vi "Matrix - Complex.vi"(5 "use temporary file?":bool, 7 "data type of variable":cdb[][](array[numeric]), 8 "error in":errorcluster, 10 "variable name":string, 11 "pipe in":T1) -> (0 "error out":errorcluster, 2 "value":cdb[][](array[numeric]) format="%.2f", 3 "pipe out":T1)   [LabVIEW 2013, in "GOLPI library.lvlib"]
uses:
  GOLPI library.lvlib
  LV Process.lvlibp/Pipe Handle.ctl
  Custom Error Codes Enum Type Def.vi
  LV Process.lvlibp
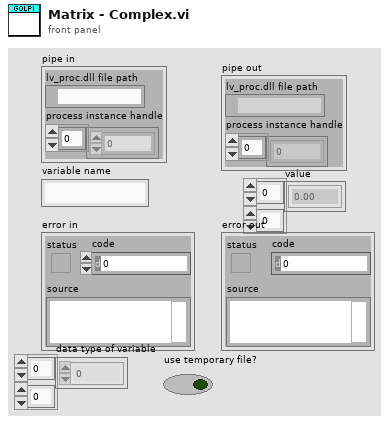
[diagram p1: front panel]
types:
  T1 = typedef "LV Process.lvlibp/Pipe Handle.ctl" = cluster{"lv_proc.dll file path":path, "process instance handle":u32[]}
  T2 = typedef "GOLPI library.lvlib/Custom Error Codes Enum Type Def.vi" = enum16{"no error", "00 working directory PAR1 missing", "01 octave binary PAR1 missing", "02 octave report error PAR1", "03 empty output last cmd PAR1", "04 missing temporary file PAR1", "10 var PAR1 not string", "11 var PAR1 not num, scal, ~compl", "12 var PAR1 not num, scal, compl", "13 var PAR1 not num, vect, ~compl", "14 var PAR1 not num, vect, compl", "15 var PAR1 not num, mat, ~compl", "16 var PAR1 not num, mat, ~compl", "99 not finished"}
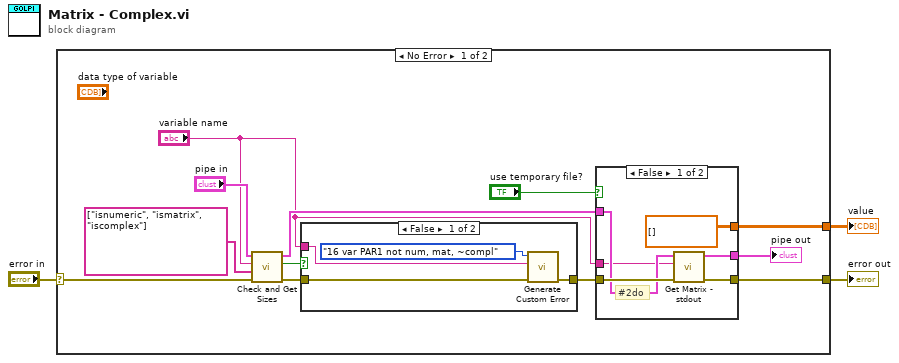
[diagram p0: block diagram]
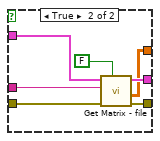
[diagram p2: hidden frame]
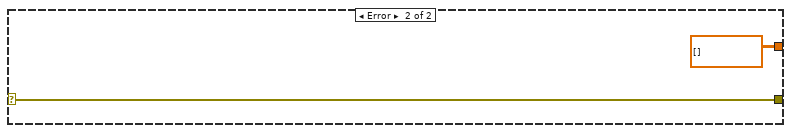
[diagram p4: hidden frame]
diagram:
  n1 = case shown="No Error" "error in" {
    selector: "error in" -> [w13 w35]
    tunnel: [w7 w35] -> w3
    tunnel: [w4 cdb[][] [] ("value")] -> w1
    frame No Error {
      n2 = call "Check and Get Sizes.vi"("error in (no error)"=w13, "test commands"=string[] ["isnumeric", "ismatrix", "iscomplex"], "variable name"="variable name", "pipe in"="pipe in") -> ("error out"=w12:errorcluster, "all tests OK?"=w14:bool, "pipe out"=w10:T1)  [unwired: 4 in, 1 out]
      n3 = case shown="False" w14 {
        tunnel: w12 -> [w31 w33]
        tunnel: [w30 w33] -> w8
        tunnel: "variable name" -> [w29 _]
        frame False {
          n4 = call "Generate Custom Error.vi"("error in"=w31, "PAR1"=w29, "Enum"=Custom_Error_Codes_Enum_Type_Def.vi."16 var PAR1 not num, mat, ~compl") -> ("error out"=w30:errorcluster)  [unwired: 8 in]
        }
        frame True {
        }
      }
      n5 = case shown="False" "use temporary file?" {
        tunnel: w10 -> [w18 w24]
        tunnel: [w17 w25] -> w9
        tunnel: w8 -> [w20 w27]
        tunnel: [w19 w26] -> w7
        tunnel: "variable name" -> [w16 w23]
        tunnel: [cdb[][] [] ("value") w22] -> w4
        frame False {
          # "#2do"
          n6 = call "Get Matrix - stdout.vi"("error in (no error)"=w20, "variable name"=w16, "pipe in"=w18) -> ("error out"=w19:errorcluster, "pipe out"=w17:T1)  [unwired: 6 in, 1 out]
        }
        frame True {
          n7 = call "Get Matrix - file.vi"("is string"=FALSE, "error in (no error)"=w27, "variable name"=w23, "pipe in"=w24) -> ("error out"=w26:errorcluster, "cmplx double array"=w22:cdb[][], "pipe out"=w25:T1)  [unwired: 3 in, 2 out]
        }
      }
      "pipe out" <- w9
    }
    frame Error {
    }
  }
  "value" <- w1
  "error out" <- w3
